vi "Get Transfer Buffers.vi"(8 "error in":errorcluster, 10 "buffer descriptor":T1, 11 "buffers":T3) -> (0 "error out":errorcluster, 2 "status":refnum<class "Status Pointer.lvclass">, 3 "buffer":refnum<class "Buffer.lvclass">)   [LabVIEW 2021, in "DSF Core.lvlib" / "Data Server Thread.lvclass"]
uses:
  Data Server Thread.lvclass
  Buffer/Buffer.lvclass
  C:/Program Files/National Instruments/LabVIEW 2021/vi.lib/NI/Memory Manager/Classes/Pointer/Pointer.lvclass
  Framework.ctl
  Buffers/Buffers.lvclass
  Status/Status Pointer.lvclass
  Plugin.ctl
  Group.ctl
  Transfer/Transfer.lvclass
  DSF Buffer Subset Descriptor.ctl
  Typedefs/DSF Buffer Type.ctl
  Transfer/Transfer.lvclass/Transfer.ctl
  Buffers/Buffers.lvclass/Buffers.ctl
  <vilib>/NI/Memory Manager/Classes/Pointer/Pointer.lvclass/Pointer.ctl
  Buffers/Get Active Buffers.vi
  <vilib>/NI/Memory Manager/Classes/Pointer/Get Address.vi
  <vilib>/NI/Memory Manager/Classes/Pointer/Encapsulate.vi
  <vilib>/NI/Memory Manager/Classes/Pointer/Check Null Pointer.vi
  <vilib>/NI/Memory Manager/Classes/Pointer/Check Length.vi
  <vilib>/NI/Memory Manager/Classes/Pointer/Set Size.vi
  <vilib>/NI/Memory Manager/Classes/Pointer/Set Address.vi
  <vilib>/NI/Memory Manager/Classes/Pointer/Set Internal.vi
  <vilib>/NI/Memory Manager/Classes/Pointer/Errors.vi
  <vilib>/NI/Memory Manager/Classes/Pointer/Null Pointer.vi
  <vilib>/NI/Memory Manager/Classes/Pointer/Is Null.vi
  <vilib>/NI/Memory Manager/Classes/Pointer/Get Size.vi
  <vilib>/NI/Memory Manager/Classes/Pointer/Check Bounds (Pointer).vi
  <vilib>/NI/Memory Manager/Classes/Pointer/Create Error.vi
  <vilib>/NI/Memory Manager/Classes/Pointer/Out of Bounds.vi
  <vilib>/NI/Memory Manager/VIs/New Error Cluster.vi
  <vilib>/NI/Memory Manager/VIs/New Error Cluster (512B).vi
  <vilib>/NI/Memory Manager/VIs/Set Error Status.vi
  <vilib>/NI/Memory Manager/VIs/Set Error Code.vi
  <vilib>/NI/Memory Manager/VIs/Set Error Source.vi
  <vilib>/NI/Memory Manager/Constants/Constants.vi
  <vilib>/NI/Memory Manager/Constants/Library Name.vi
  <vilib>/NI/Memory Manager/Classes/Pointer/Pointer Error Info.vi
  <vilib>/NI/Memory Manager/VIs/Write String to Source.vi
  <vilib>/NI/Memory Manager/Constants/Pointer Class Name.vi
  <vilib>/NI/Memory Manager/Classes/Pointer/Write Pointer Size to Error.vi
  <vilib>/NI/Memory Manager/VIs/Write Numeric to Source.vi
  <vilib>/NI/Memory Manager/VIs/Write Numeric Scalar to Source (Base10 U64).vi
  <vilib>/NI/Memory Manager/Classes/Pointer/Pointer.lvclass
  DSF Core.lvlib
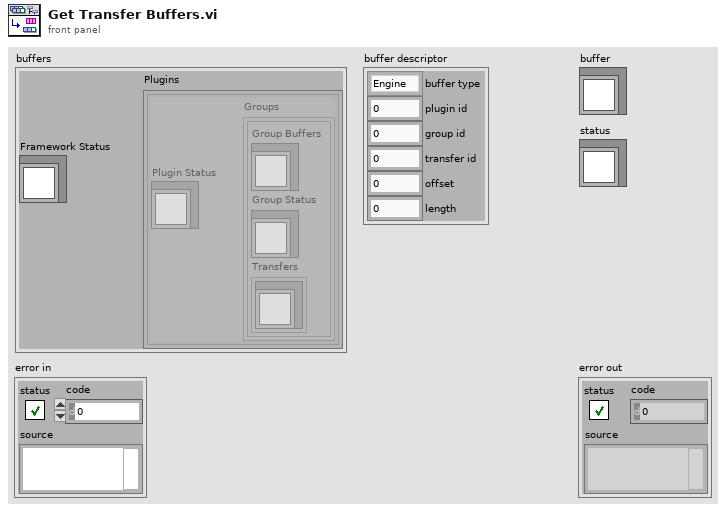
[diagram p1: front panel]
types:
  T1 = typedef "DSF Core.lvlib/DSF Buffer Subset Descriptor.ctl" = cluster{"buffer type":T2, "plugin id":i32, "group id":i32, "transfer id":i32, "offset":u64, "length":i64}
  T2 = typedef "DSF Core.lvlib/DSF Buffer Type.ctl" = enum16{"Engine", "String"}
  T3 = typedef "DSF Core.lvlib/Data Server Thread.lvclass/Framework.ctl" = cluster{"Framework Status":refnum<class "Status Pointer.lvclass">, "Plugins":T4[]}
  T4 = typedef "DSF Core.lvlib/Data Server Thread.lvclass/Plugin.ctl" = cluster{"Plugin Status":refnum<class "Status Pointer.lvclass">, "Groups":T5[]}
  T5 = typedef "DSF Core.lvlib/Data Server Thread.lvclass/Group.ctl" = cluster{"Group Buffers":refnum<class "Buffers.lvclass">, "Group Status":refnum<class "Status Pointer.lvclass">, "Transfers":refnum<class "Transfer.lvclass">[]}
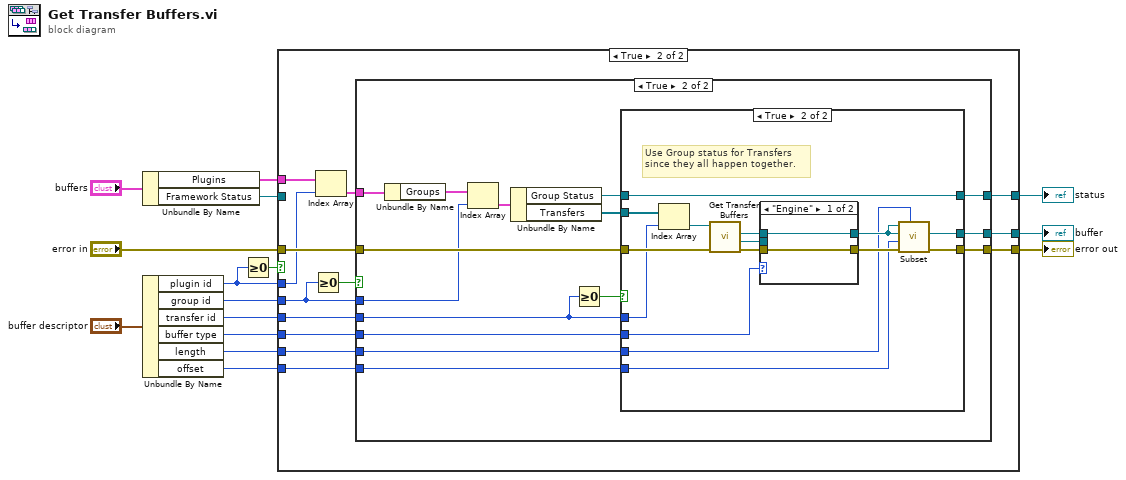
[diagram p0: block diagram]
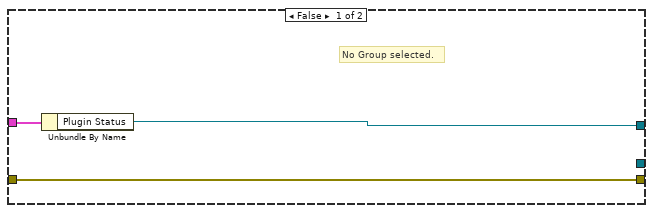
[diagram p3: hidden frame]
diagram:
  n1 = Unbundle By Name("buffers") -> ("Plugins"=w2:T4[], "Framework Status"=w1:refnum<class "Status Pointer.lvclass">)
  n2 = Unbundle By Name("buffer descriptor") -> ("plugin id"=w7:i32, "group id"=w12:i32, "transfer id"=w11:i32, "buffer type"=w3:T2, "length"=w14:i64, "offset"=w10:u64)
  n3 = Greater Or Equal To 0?(x=w7) -> (x >= 0?=w6:bool)
  n4 = case shown="True" w6 {
    tunnel: "error in" -> [w17 w30]
    tunnel: w14 -> [_ w29]
    tunnel: w12 -> [_ w22]
    tunnel: w11 -> [_ w28]
    tunnel: w10 -> [_ w27]
    tunnel: [w17 w26] -> w9
    tunnel: [_ w25] -> w8
    tunnel: w7 -> [_ w24]
    tunnel: [w16 w21] -> w5
    tunnel: w3 -> [_ w20]
    tunnel: w2 -> [_ w19]
    tunnel: w1 -> [w16 _]
    frame False {
      # "No Plugin selected."
    }
    frame True {
      n5 = Greater Or Equal To 0?(x=w22) -> (x >= 0?=w23:bool)
      n6 = Index Array(array=w19, index=w24) -> (element=w18:T4)
      n7 = case shown="True" w23 {
        tunnel: w18 -> [w31 w48]
        tunnel: w30 -> [w33 w46]
        tunnel: w29 -> [_ w45]
        tunnel: w28 -> [_ w40]
        tunnel: w27 -> [_ w44]
        tunnel: [w33 w43] -> w26
        tunnel: [_ w42] -> w25
        tunnel: w22 -> [_ w41]
        tunnel: [w32 w38] -> w21
        tunnel: w20 -> [_ w37]
        frame False {
          # "No Group selected."
          n8 = Unbundle By Name(w31) -> ("Plugin Status"=w32:refnum<class "Status Pointer.lvclass">)
        }
        frame True {
          n9 = Unbundle By Name(w48) -> ("Groups"=w47:T5[])
          n10 = Index Array(array=w47, index=w41) -> (element=w36:T5)
          n11 = Unbundle By Name(w36) -> ("Group Status"=w35:refnum<class "Status Pointer.lvclass">, "Transfers"=w34:refnum<class "Transfer.lvclass">[])
          n12 = Greater Or Equal To 0?(x=w40) -> (x >= 0?=w39:bool)
          n13 = case shown="True" w39 {
            tunnel: w46 -> [w49 w64]
            tunnel: w45 -> [_ w52]
            tunnel: w40 -> [_ w63]
            tunnel: w44 -> [_ w51]
            tunnel: [w49 w62] -> w43
            tunnel: [_ w61] -> w42
            tunnel: [w50 w54] -> w38
            tunnel: w35 -> [w50 w54]
            tunnel: w37 -> [_ w58]
            tunnel: w34 -> [_ w53]
            frame False {
              # "No Transfer selected."
            }
            frame True {
              # "Use Group status for Transfers since they all happen together."
              n14 = Index Array(array=w53, index=w63) -> (element=w65:refnum<class "Transfer.lvclass">)
              n15 = call "Get Transfer Buffers.vi"("error in (no error)"=w64, "Transfer in"=w65) -> ("error out"=w60:errorcluster, "string Buffer"=w57:refnum<class "Buffer.lvclass">, "engine Buffer"=w56:refnum<class "Buffer.lvclass">)  [unwired: 6 in, 1 out]
              n16 = case shown="\"Engine\"" w58 {
                tunnel: w60 -> [w67 w69]
                tunnel: [w67 w69] -> w59
                tunnel: w57 -> [_ w68]
                tunnel: w56 -> [w66 _]
                tunnel: [w66 w68] -> w55
                frame "Engine" {
                }
                frame "String" {
                }
              }
              n17 = call <vilib>:"Subset.vi"("length (-1: rest)"=w52, "error in (no error)"=w59, "offset (0)"=w51, "subset Pointer type"=w55, "base Pointer in"=w55) -> ("error out"=w62:errorcluster, "subset Pointer"=w61:refnum<class "Buffer.lvclass">)  [unwired: 3 in, 2 out]
            }
          }
        }
      }
    }
  }
  "error out" <- w9
  "buffer" <- w8
  "status" <- w5
